vi "ST_do_SQL_query.vi"(6 "station":T1, 8 "error_in":errorcluster, 10 "SQL_query":string, 11 "SQL_connection_reference":T2) -> (0 "error_out":errorcluster, 3 "recordset_out":variant[][](array[variant]))   [LabVIEW 2020]
uses:
  <vilib>/addons/database/Connection.llb/Conn ObjectReference.ctl
  station.ctl
  FGV/DIAGNOSTICS_message_history_buffer/FGV_PROXY_DIAGNOSTICS_message_history_buffer.ctl
  <vilib>/addons/database/Connection.llb/Conn Execute.vi
  <vilib>/addons/database/Recordset.llb/Rec Fetch Recordset Data (R).vi
  <vilib>/addons/database/Recordset.llb/Rec Destroy - Connection.vi
  <vilib>/addons/database/NI_Database_API.lvlib
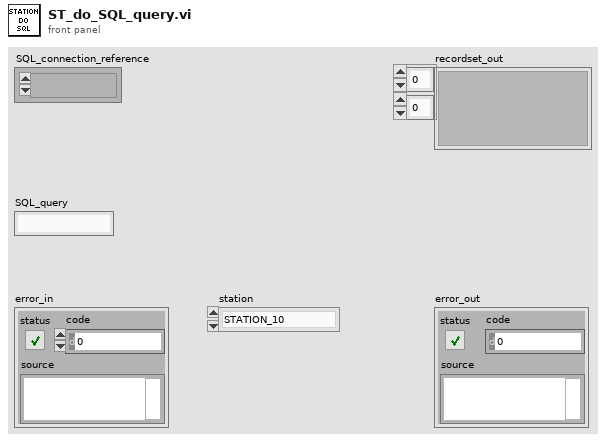
[diagram p1: front panel]
types:
  T1 = typedef "station.ctl" = enum16{"STATION_10", "STATION_20", "STATION_30", "STATION_40", "STATION_50", "STATION_60", "STATION_70", "STATION_80", "STATION_90", "STATION_100", "STATION_110", "STATION_120", "STATION_165", "MAIN"}
  T2 = typedef "NI_Database_API.lvlib/Conn ObjectReference.ctl" = refnum<k1>
  T3 = typedef "FGV_PROXY_DIAGNOSTICS_message_history_buffer.ctl" = enum16{"initialize", "add_TCP_PLC_to_PC", "add_TCP_PC_to_PLC", "add_SQL_PC_to_DB", "add_SQL_transaction", "add_SQL_DB_to_PC", "get_station", "get_all", "clear_station", "clear_all", "save_log"}
  T4 = typedef "NI_Database_API.lvlib/Rec ObjectReference.ctl" = refnum<k1>
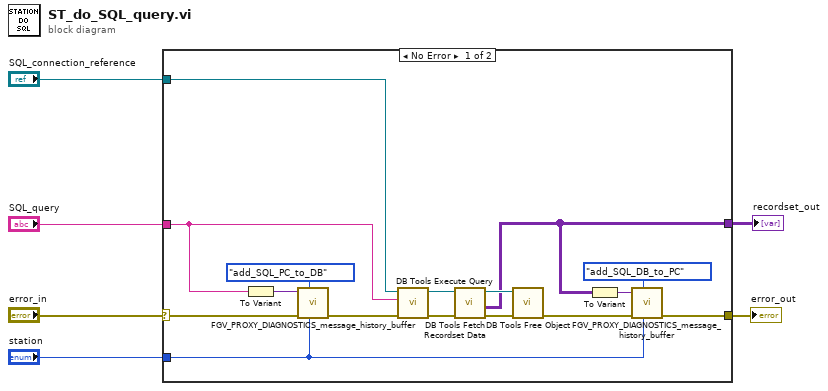
[diagram p0: block diagram]
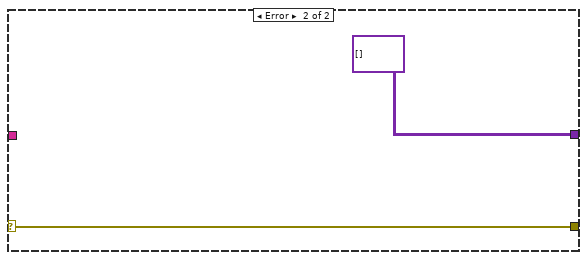
[diagram p2: hidden frame]
diagram:
  n1 = case shown="No Error" "error_in" {
    selector: "error_in" -> [w15 w24]
    tunnel: [w8 variant[][] [] ("recordset data")] -> w6
    tunnel: [w9 w24] -> w5
    tunnel: "SQL_query" -> [w13 _]
    tunnel: "SQL_connection_reference" -> [w22 _]
    tunnel: "station" -> [w7 _]
    frame No Error {
      n2 = To Variant(anything=w13) -> (Variant=w17:variant)
      n3 = call "FGV_PROXY_DIAGNOSTICS_message_history_buffer.vi"("station"=w7, "options"=FGV_PROXY_DIAGNOSTICS_message_history_buffer."add_SQL_PC_to_DB", "error_in"=w15, "input"=w17) -> ("error_out"=w14:errorcluster)  [unwired: 6 in, 1 out]
      n4 = call-poly <vilib>:"DB Tools Execute Query.vi"("error in (no error)"=w14, "SQL query"=w13, "connection reference"=w22) -> ("error out"=w20:errorcluster, "recordset reference"=w19:T4)  [unwired: 5 in]
      n5 = call-poly <vilib>:"DB Tools Fetch Recordset Data.vi"("error in (no error)"=w20, "recordset reference"=w19) -> ("error out"=w21:errorcluster, "recordset data"=w8:variant[][], "recordset reference out"=w18:T4)  [unwired: 3 in]
      n6 = call-poly <vilib>:"DB Tools Free Object.vi"("error in (no error)"=w21, "recordset reference"=w18) -> ("error out"=w10:errorcluster)  [unwired: 8 in, 1 out]
      n7 = To Variant(anything=w8) -> (Variant=w11:variant)
      n8 = call "FGV_PROXY_DIAGNOSTICS_message_history_buffer.vi"("station"=w7, "options"=FGV_PROXY_DIAGNOSTICS_message_history_buffer."add_SQL_DB_to_PC", "error_in"=w10, "input"=w11) -> ("error_out"=w9:errorcluster)  [unwired: 6 in, 1 out]
    }
    frame Error {
    }
  }
  "recordset_out" <- w6
  "error_out" <- w5
